vi "Connect.vi"(8 "error in (no error)":errorcluster, 11 "NRT8000 in":refnum<class "NRT8000.lvclass">) -> (0 "error out":errorcluster, 3 "NRT8000 out":refnum<class "NRT8000.lvclass">)   [LabVIEW 2018, in "NRT8000.lvlib" / "NRT8000.lvclass"]
uses:
  NRT8000.lvclass
  PPLs/Optical Spectrum Analyzer/Parent/OSA.lvlibp/Optical Spectrum Analyzer.lvclass
  <vilib>/Instr/_visa.llb/VISA Configure Serial Port (Instr).vi
  C:/Projects/LabVIEW/PPLs/Optical Spectrum Analyzer/Parent/OSA.lvlibp/Optical Spectrum Analyzer.lvclass
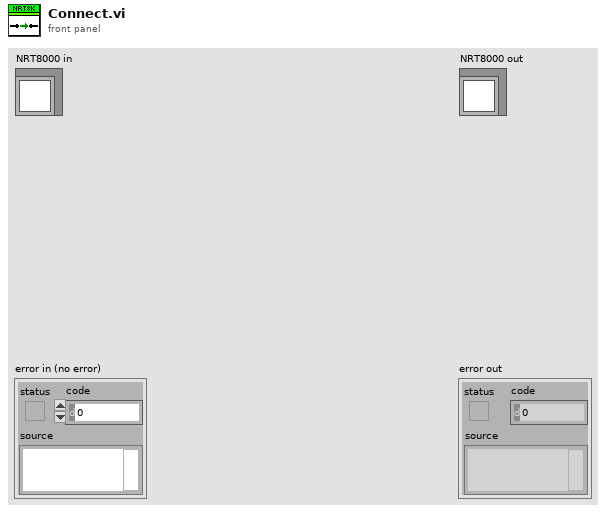
[diagram p1: front panel]
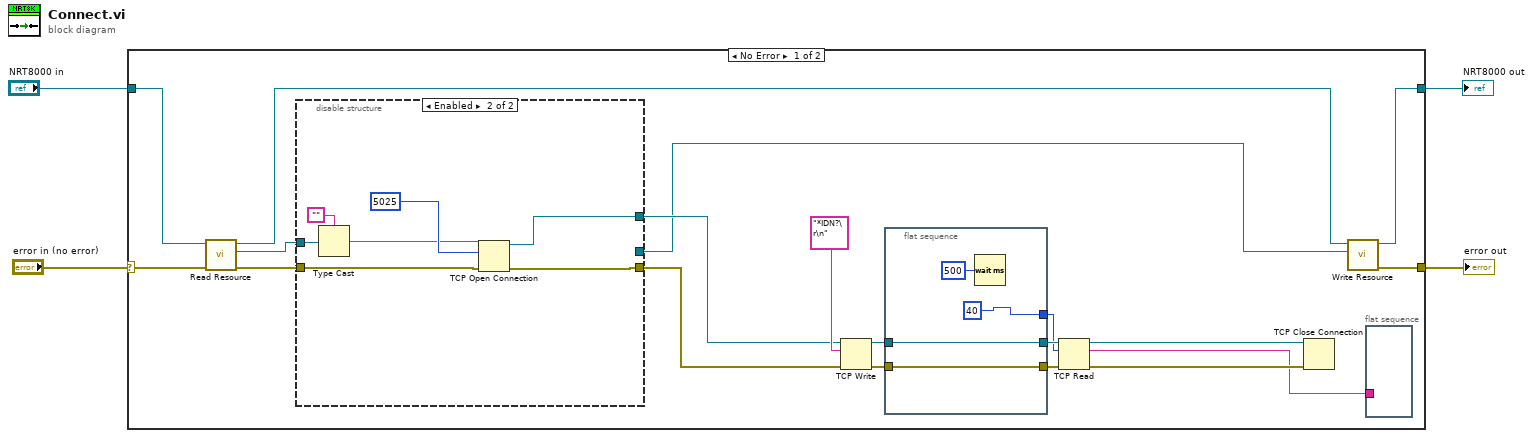
[diagram p0: block diagram]
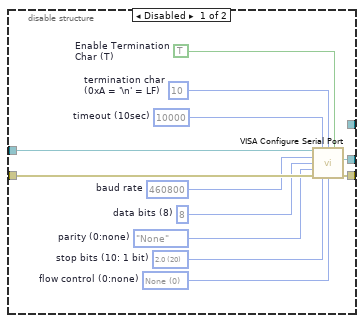
[diagram p2: hidden frame]
diagram:
  n1 = case shown="No Error" "error in (no error)" {
    selector: "error in (no error)" -> [w23 w48]
    tunnel: [w18 w48] -> w3
    tunnel: "NRT8000 in" -> [w22 w47]
    tunnel: [w17 w47] -> w1
    frame No Error {
      n2 = call "Read Resource.vi"("error in (no error)"=w23, "Optical Spectrum Analyzer in"=w22) -> ("error out"=w21:errorcluster, "Resource"=w20:refnum<visa-resource-name>, "Optical Spectrum Analyzer out"=w19:refnum<class "NRT8000.lvclass">)  [unwired: 7 in]
      n3 = disable-structure shown="Enabled" {
        disable-tunnel: w21 -> [w39 w42]
        disable-tunnel: w20 -> [w38 w46]
        disable-tunnel: [w29 _] -> w5
        disable-tunnel: [w28 w40] -> w11
        disable-tunnel: [_ w41] -> w12
        frame Disabled {
          w30 = TRUE  # Enable Termination Char (T)
          w31 = u8 10  # termination char (0xA = '\n' = LF)
          w32 = u32 10000  # timeout (10sec)
          w33 = u16 0 items=["None", "XON/XOFF", "RTS/CTS", "XON/XOFF & RTS/CTS", "DTR/DSR", "XON/XOFF & DTR/DSR"]  # flow control (0:none)
          w34 = u16 20 items=["1.0"=10, "1.5"=15, "2.0"=20]  # stop bits (10: 1 bit)
          w35 = enum16{"None", "Odd", "Even", "Mark", "Space"}."None"  # parity (0:none)
          w36 = u16 8  # data bits (8)
          w37 = u32 460800  # baud rate
          n4 = call-poly "VISA Configure Serial Port"("VISA resource name"=w38, "timeout (10sec)"=w32, "termination char\n(0xA = '\\n' = LF)"=w31, "Enable Termination\nChar (T)"=w30, "baud rate (9600)"=w37, "data bits (8)"=w36, "parity (0:none)"=w35, "error in (no error)"=w39, "stop bits (10: 1 bit)"=w34, "flow control (0:none)"=w33) -> ("VISA resource name out"=w29:refnum<visa-resource-name>, "error out"=w28:errorcluster)  [unwired: 4 in]
        }
        frame Enabled {
          n5 = Type Cast(type="", x=w46) -> (*(type *) &x=w43:string)
          n6 = TCP Open Connection(address=w43, remote port or service name=u16 5025 ("local port (0)"), error in (no error)=w42) -> (connection ID=w41:refnum<k5>, error out=w40:errorcluster)  [unwired: 2 in]
        }
      }
      n7 = TCP Write(connection ID=w12, data in="*IDN?\r\n", error in (no error)=w11) -> (connection ID out=w9:refnum<k5>, error out=w8:errorcluster)  [unwired: 1 in, 1 out]
      n8 = flat-sequence {
        tunnel: [w27] -> w10
        tunnel: w9 -> [w27]
        tunnel: w8 -> [w26]
        tunnel: [w26] -> w7
        tunnel: [40] -> w6
        frame #0 {
          n9 = Wait (ms)(milliseconds to wait=u32 500) -> ()  [unwired: 1 out]
        }
      }
      n10 = TCP Read(connection ID=w10, bytes to read=w6, error in (no error)=w7) -> (connection ID out=w15:refnum<k5>, data out=w13:string, error out=w14:errorcluster)  [unwired: 2 in]
      n11 = TCP Close Connection(connection ID=w15, error in (no error)=w14) -> ()  [unwired: 1 in, 2 out]
      n12 = call "Write Resource.vi"("Resource"=w5, "Optical Spectrum Analyzer in"=w19) -> ("error out"=w18:errorcluster, "Optical Spectrum Analyzer out"=w17:refnum<class "NRT8000.lvclass">)  [unwired: 8 in]
      n13 = flat-sequence {
        tunnel: w13 -> [_]
        frame #0 {
        }
      }
    }
    frame Error {
    }
  }
  "error out" <- w3
  "NRT8000 out" <- w1
